vi "Reset Gyro Angle.vi"(8 "error in":errorcluster, 11 "Reset":bool) -> (0 "error out":errorcluster)   [LabVIEW 2016, in "Path Track.lvlib"]
uses:
  Path Track.lvlib
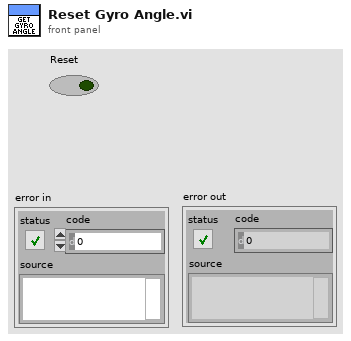
[diagram p1: front panel]
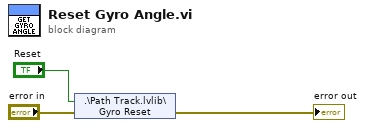
[diagram p0: block diagram]
diagram:
  n1 = shared-variable ".\\Path Track.lvlib\\Gyro Reset"("Reset", error in="error in") -> (error out=→"error out":errorcluster)
